vi "main  1.0.vi"() -> ()   [LabVIEW 2018]
uses:
  <vilib>/Analysis/baseanly.llb/Mean (DBL).vi
  <vilib>/Instr/_visa.llb/VISA Configure Serial Port (Instr).vi
  <vilib>/Analysis/NI_AALBase.lvlib
panel:
  out "提示":string
  out "错误指示":bool
  in  "单片机COM":refnum<visa-resource-name>
  out "上一路数据图":dbl[](graph)
  in  "数据存储位置":path
  in  "开关":bool
  out "2-7 2":bool
  out "2-6 2":bool
  out "2-5 2":bool
  out "2-4 2":bool
  out "2-3 2":bool
  out "2-2 2":bool
  out "2-1 2":bool
  out "1-7 2":bool
  out "1-6 2":bool
  out "1-5 2":bool
  out "1-4 2":bool
  out "1-3 2":bool
  out "1-2 2":bool
  out "1-1 2":bool
  out "字符串":string
  in  "1-7":bool
  in  "2-7":bool
  in  "2-6":bool
  in  "2-5":bool
  in  "2-4":bool
  in  "2-3":bool
  in  "2-2":bool
  in  "2-1":bool
  in  "1-1":bool
  in  "1-2":bool
  in  "1-3":bool
  in  "1-4":bool
  in  "1-5":bool
  in  "1-6":bool
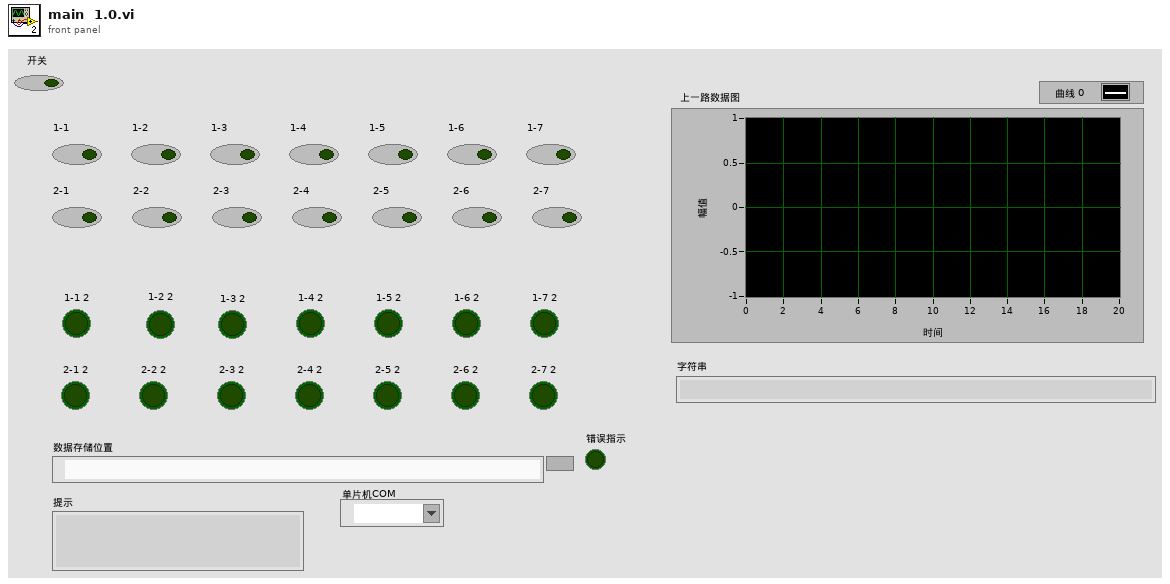
[diagram p1: front panel]
types:
  T1 = enum16{"open", "replace", "create", "open or create", "replace or create", "replace or create with confirmation"}
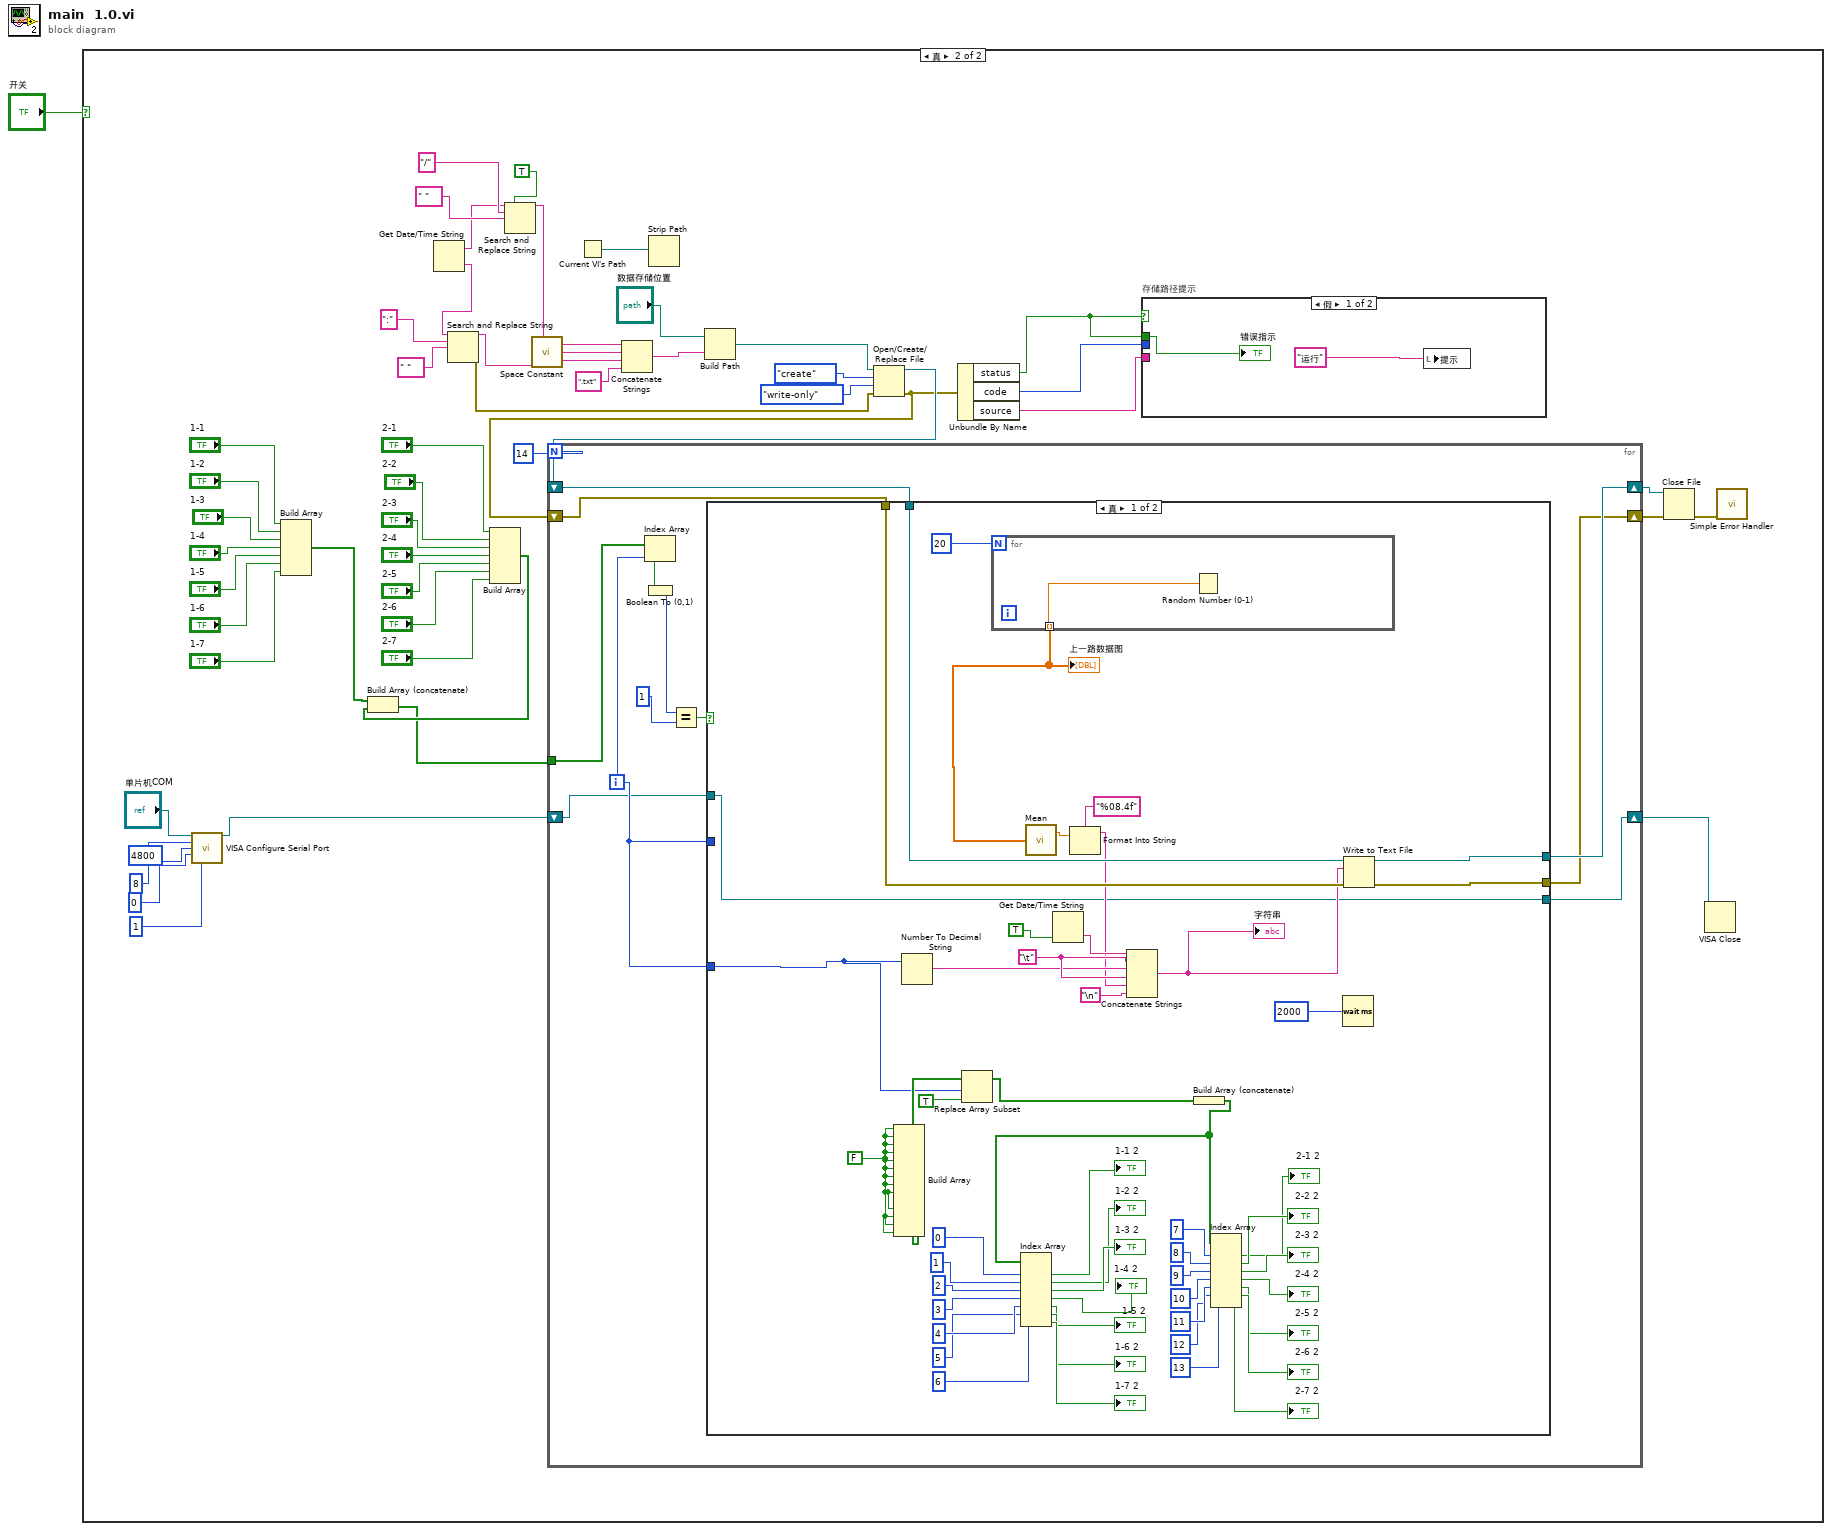
[diagram p0: block diagram]
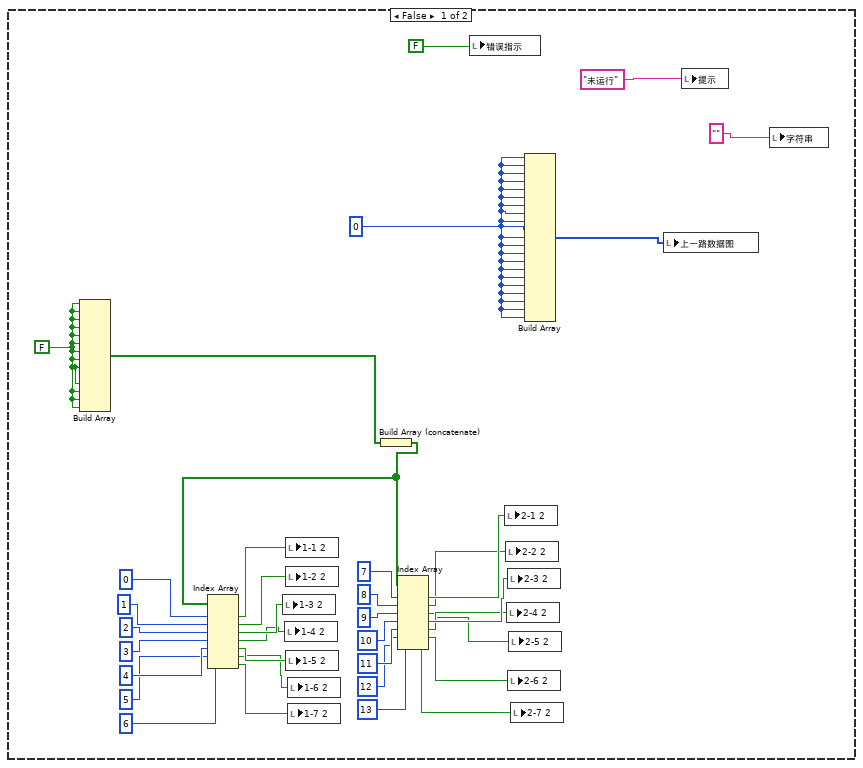
[diagram p2: hidden frame]
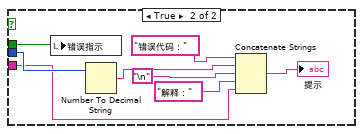
[diagram p3: hidden frame]
diagram:
  n1 = case shown="真" "开关" {
    frame False {
      w5 = 0
      w37 = FALSE
      n2 = Build Array(w37, w37, w37, w37, w37, w37, w37, w37, w37, w37, w37, w37, w37, w37) -> (w21:bool[])
      n3 = Build Array (concatenate)(w21) -> (w36:bool[])
      n4 = Index Array(array=w36, index #1=0, index #2=1, index #3=2, index #4=3, index #5=4, index #6=5, index #7=6) -> (element #1=w13:bool, element #2=w12:bool, element #3=w11:bool, element #4=w10:bool, element #5=w9:bool, element #6=w8:bool, element #7=w7:bool)
      n5 = local write "1-3 2"(w11) -> ()
      n6 = local write "1-4 2"(w10) -> ()
      n7 = local write "1-1 2"(w13) -> ()
      n8 = local write "1-2 2"(w12) -> ()
      n9 = local write "1-5 2"(w9) -> ()
      n10 = local write "1-6 2"(w8) -> ()
      n11 = local write "1-7 2"(w7) -> ()
      n12 = Index Array(array=w36, index #1=7, index #2=8, index #3=9, index #4=10, index #5=11, index #6=12, index #7=13) -> (element #1=w20:bool, element #2=w19:bool, element #3=w16:bool, element #4=w18:bool, element #5=w17:bool, element #6=w15:bool, element #7=w14:bool)
      n13 = local write "错误指示"(FALSE) -> ()
      n14 = local write "2-1 2"(w20) -> ()
      n15 = local write "2-2 2"(w19) -> ()
      n16 = local write "2-4 2"(w17) -> ()
      n17 = local write "2-3 2"(w18) -> ()
      n18 = local write "2-6 2"(w15) -> ()
      n19 = local write "2-5 2"(w16) -> ()
      n20 = local write "2-7 2"(w14) -> ()
      n21 = Build Array(w5, w5, w5, w5, w5, w5, w5, w5, w5, w5, w5, w5, w5, w5, w5, w5, w5, w5, w5, w5, w5) -> (w6:i32[])
      n22 = local write "上一路数据图"(w6) -> ()
      n23 = local write "提示"("未运行") -> ()
      n24 = local write "字符串"("") -> ()
    }
    frame True {
      n25 = call-poly "VISA Configure Serial Port"("VISA resource name"="单片机COM", "baud rate (9600)"=4800, "data bits (8)"=8, "parity (0:none)"=0, "stop bits (10: 1 bit)"=1) -> ("VISA resource name out"=w42:refnum<visa-resource-name>)  [unwired: 9 in, 1 out]
      n26 = Build Array("1-1", "1-2", "1-3", "1-4", "1-5", "1-6", "1-7") -> (w74:bool[])
      n27 = Get Date/Time String() -> (date string=w56:string, time string=w63:string)  [unwired: 3 in]
      n28 = Search and Replace String(input string=w63, search string=":", replace string=" ") -> (result string=w53:string, error out=w60:errorcluster)  [unwired: 5 in, 2 out]
      n29 = Build Array("2-1", "2-2", "2-3", "2-4", "2-5", "2-6", "2-7") -> (w73:bool[])
      n30 = Build Array (concatenate)(w74, w73) -> (w72:bool[])
      n31 = Search and Replace String(replace all?=TRUE, input string=w56, search string="/", replace string=" ") -> (result string=w55:string)  [unwired: 4 in, 3 out]
      n32 = call <vilib>:"Space Constant.vi"() -> ("String"=w59:string)
      n33 = Current VI's Path() -> (path=w66:path)
      n34 = Concatenate Strings(w55, w59, w53, ".txt") -> (w70:string)
      n35 = Strip Path(path=w66) -> ()  [unwired: 2 out]
      n36 = Build Path(base path="数据存储位置", name or relative path=w70) -> (appended path=w65:path)
      n37 = Open/Create/Replace File(file path (use dialog)=w65, error in=w60, operation (0:open)=T1."create", access (0:read/write)=enum16{"read/write", "read-only", "write-only"}."write-only") -> (refnum out=w67:refnum<file>, error out=w41:errorcluster)  [unwired: 3 out]
      n38 = for {
        N: 14 -> [_]
        tunnel: w72 -> [w102]
        shift-right: [w106] -> w51
        shift-left: w67 -> [w104]
        shift-right: [w105] -> w52
        shift-left: w41 -> [w103]
        shift-right: [w99] -> w43
        shift-left: w42 -> [w100]
        i -> [w101]
        n39 = Index Array(array=w102, index=w101) -> (element=w110:bool)
        n40 = Boolean To (0,1)(Boolean=w110) -> (0, 1=w108:i16)
        n41 = Equal?(x=w108, y=1) -> (x = y?=w107:bool)
        n42 = case shown="真" w107 {
          tunnel: w104 -> [w160 w164]
          tunnel: w101 -> [w112 _]
          tunnel: [w156 w164] -> w106
          tunnel: [w117 w165] -> w105
          tunnel: w103 -> [w154 w165]
          tunnel: w100 -> [w111 w163]
          tunnel: w101 -> [_ _]
          tunnel: [w111 w163] -> w99
          frame True {
            w150 = FALSE
            w157 = "\t" ("Tab")
            n43 = Build Array(w150, w150, w150, w150, w150, w150, w150, w150, w150, w150, w150, w150, w150, w150) -> (w149:bool[])
            n44 = Number To Decimal String(number=w112) -> (decimal integer string=w153:string)  [unwired: 1 in]
            n45 = Replace Array Subset(array=w149, new element=TRUE, index=w112) -> (w118:bool[])
            n46 = for {
              N: 20 -> [_]
              tunnel: [w162] -> w115 mode=indexing
              n47 = Random Number (0-1)() -> (number: 0 to 1=w162:dbl)
            }
            "上一路数据图" <- w115
            n48 = call-poly <vilib>:"Mean.vi"("X"=w115) -> ("mean"=w114:dbl)  [unwired: 1 out]
            n49 = Get Date/Time String(want seconds? (F)=TRUE) -> (time string=w158:string)  [unwired: 2 in, 1 out]
            n50 = Format Into String(format string="%08.4f" ("格式字符串"), w114) -> (resulting string=w113:string)  [unwired: 2 in, 1 out]
            n51 = Concatenate Strings(w158, w157, w153, w157, w113, "\n") -> (w152:string)
            "字符串" <- w152
            n52 = Build Array (concatenate)(w118) -> (w133:bool[])
            n53 = Index Array(array=w133, index #1=0, index #2=1, index #3=2, index #4=3, index #5=4, index #6=5, index #7=6) -> (element #1=→"1-1 2":bool, element #2=→"1-2 2":bool, element #3=→"1-3 2":bool, element #4=→"1-4 2":bool, element #5=→"1-5 2":bool, element #6=→"1-6 2":bool, element #7=→"1-7 2":bool)
            n54 = Index Array(array=w133, index #1=7, index #2=8, index #3=9, index #4=10, index #5=11, index #6=12, index #7=13) -> (element #1=→"2-1 2":bool, element #2=→"2-2 2":bool, element #3=→"2-3 2":bool, element #4=→"2-4 2":bool, element #5=→"2-5 2":bool, element #6=→"2-6 2":bool, element #7=→"2-7 2":bool)
            n55 = Wait (ms)(milliseconds to wait=u32 2000) -> ()  [unwired: 1 out]
            n56 = Write to Text File(file (use dialog)=w160, text=w152, error in=w154) -> (refnum out=w156:refnum<file>, error out=w117:errorcluster)  [unwired: 1 in, 1 out]
          }
          frame False {
          }
        }
      }
      n57 = Unbundle By Name(w41) -> ("status"=w38:bool, "code"=w40:i32, "source"=w39:string)
      n58 = case "存储路径提示" shown="假" w38 {
        tunnel: w40 -> [_ w97]
        tunnel: w39 -> [_ w92]
        tunnel: w38 -> [w90 w98]
        frame False {
          n59 = local write "提示"("运行") -> ()
          "错误指示" <- w90
        }
        frame True {
          n60 = local write "错误指示"(w98) -> ()
          n61 = Number To Decimal String(number=w97) -> (decimal integer string=w95:string)  [unwired: 1 in]
          n62 = Concatenate Strings("错误代码：", w95, "\n", "解释：", w92) -> (→"提示":string)
        }
      }
      n63 = Close File(refnum=w51, error in=w52) -> (error out=w50:errorcluster)  [unwired: 1 out]
      n64 = VISA Close(VISA resource name=w43) -> ()  [unwired: 1 in, 1 out]
      n65 = call <vilib>:"Simple Error Handler.vi"("error in (no error)"=w50) -> ()  [unwired: 2 in, 7 out]
    }
  }
